vi "FTW-Logger-Construct.vi"(0 "Initialization Sequence":string, 5 "Logger Configuration":T1, 11 "error in":errorcluster) -> (4 "FTW Logger":refnum<class "FTW-Logger-Core.lvclass">, 6 "Incoming Requests":refnum<event-registration>, 15 "error out":errorcluster)   [LabVIEW 2012, in "FTW-Actor.lvlib" / "FTW-Logger-Core.lvclass"]
uses:
  FTW-Logger-Core.lvclass
  Utility/FTW-Actor-Configuration.ctl
  Message/Request/FTW-Message-IncomingRequest.lvclass
  FTW-Logger-Core.lvclass/FTW-Logger-Core.ctl
  <instcachedir>/0/FTW-JSON-ToLabVIEW_0E3E72F634BF4A9AB33E22111E055A26.lvgen/FTW-JSON-ToLabVIEW_0E3E72F634BF4A9AB33E22111E055A26_004.vi
  Core/JSON/FTW-JSON-RegexParse.vi
  Core/Regex/FTW-Regex.vi
  Core/JSON/FTW-JSON-RegexHeader.vi
  Core/Error/FTW-ERR-ThrowError.vi
  Core/Error/FTW-ERR-ThrowGenericError.vi
  Core/Container/FTW-Container-Construct.vi
  Core/Container/FTW-Container-Load-JSON.vi
  Core/Container/FTW-Container-Destroy.vi
  FTW-Actor.lvlib
panel:
  # "Inputs"
  # "Outputs"
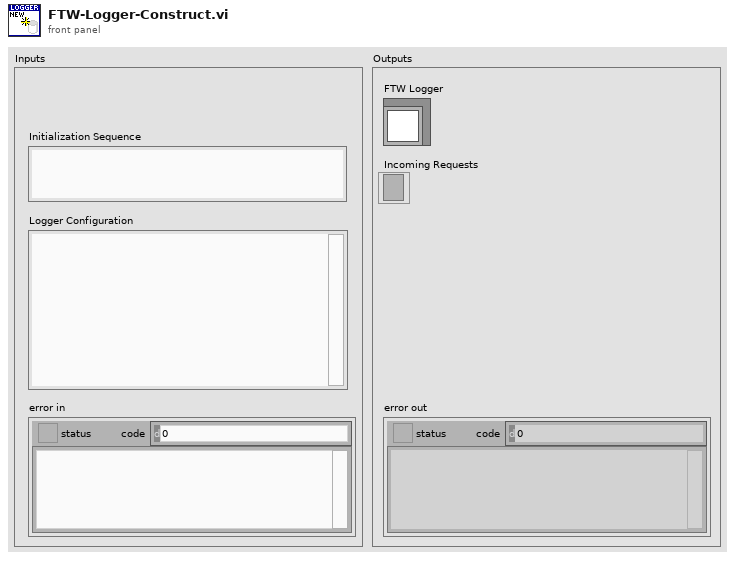
[diagram p1: front panel]
types:
  T1 = typedef "FTW-Actor.lvlib/FTW-Actor-Configuration.ctl" = string
  T2 = cluster{"LoggerDirectory":path, "LoggerDiskThrashDelay":u32, "LoggerID":string, "ApplicationName":string}
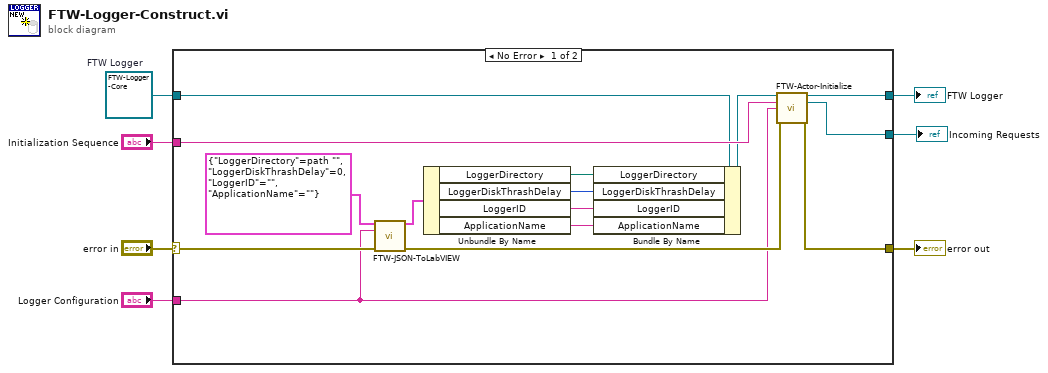
[diagram p0: block diagram]
diagram:
  w7 = refnum<class "FTW-Logger-Core.lvclass"> refnum  # FTW Logger
  n1 = case shown="No Error" "error in" {
    selector: "error in" -> [w18 w24]
    tunnel: [w20 w24] -> w5
    tunnel: [w22 w23] -> w1
    tunnel: w7 -> [w14 w23]
    tunnel: "Logger Configuration" -> [w16 _]
    tunnel: [w21 _] -> w3
    tunnel: "Initialization Sequence" -> [w19 _]
    frame No Error {
      n2 = call-generic "FTW-JSON-ToLabVIEW.vi"("Type and Defaults"=T2 {"LoggerDirectory"=path "", "LoggerDiskThrashDelay"=0, "LoggerID"="", "ApplicationName"=""}, "JSON String"=w16, "error in"=w18) -> ("Populated Values"=w12:T2, "error out"=w17:errorcluster)  [unwired: 11 in]
      n3 = Unbundle By Name(w12) -> ("LoggerDirectory"=w11:path, "LoggerDiskThrashDelay"=w10:u32, "LoggerID"=w9:string, "ApplicationName"=w8:string)
      n4 = Bundle By Name(cluster=w14, "LoggerDirectory"=w11, "LoggerDiskThrashDelay"=w10, "LoggerID"=w9, "ApplicationName"=w8) -> (w13:refnum<class "FTW-Logger-Core.lvclass">)
      n5 = call-dynamic "FTW-Actor-Initialize.vi"("FTW Actor Instance Type"=w13, "Initialization Job Sequence"=w19, "Actor Instance Configuration"=w16, "error in"=w17) -> ("FTW Actor Instance"=w22:refnum<class "FTW-Logger-Core.lvclass">, "Incoming Requests"=w21:refnum<event-registration>, "error out"=w20:errorcluster)  [unwired: 9 in]
    }
    frame Error {
    }
  }
  "error out" <- w5
  "FTW Logger" <- w1
  "Incoming Requests" <- w3
